vi "Spinner3.vi"(5 "String In":string="sweeping") -> (2 "Spinner Out":string)   [LabVIEW 2019, in "Instrument.Lockin.lvlib" / "Instrument UI.Lockin.lvclass"]
uses:
  Instrument UI.Lockin.lvclass
panel:
  out "s? t:f":i32
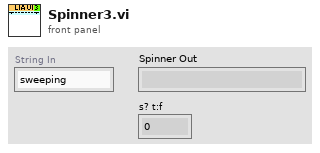
[diagram p1: front panel]
types:
  T1 = enum32{"Bad", "Idle", "Run top level", "Running"}
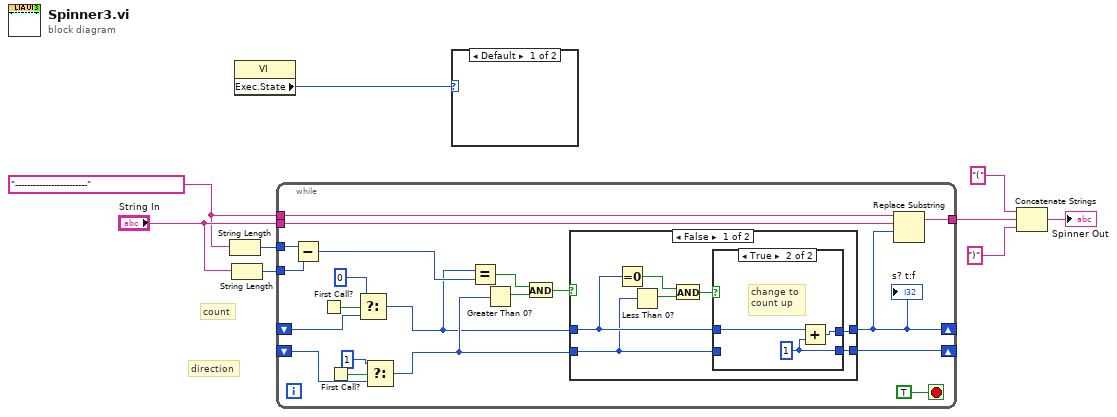
[diagram p0: block diagram]
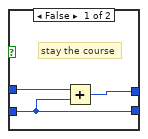
[diagram p2: hidden frame]
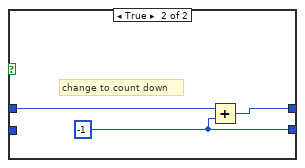
[diagram p3: hidden frame]
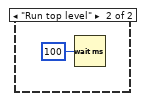
[diagram p4: hidden frame]
diagram:
  w1 = "------------------------"
  # "direction"
  # "count"
  n1 = String Length(string=w1) -> (length=w2:i32)
  n2 = String Length(string="String In") -> (length=w3:i32)
  n3 = property class="VI"() -> ("Exec.State"=w9:T1)  [unwired: 2 in, 2 out]
  n4 = while {
    tunnel: "String In" -> [w28]
    tunnel: w1 -> [w27]
    tunnel: [w26] -> w5
    shift-right: [w10] -> _
    shift-left: _ -> [w13]
    tunnel: w3 -> [w24]
    tunnel: w2 -> [w25]
    shift-right: [w19] -> _
    shift-left: _ -> [w15]
    stop <- TRUE stop-if-true
    n5 = Subtract(x=w25, y=w24) -> (x-y=w23:i32)
    n6 = First Call?() -> (First Call?: T/F=w18:bool)
    n7 = First Call?() -> (First Call?: T/F=w17:bool)
    n8 = Select(t=0 ("y"), s=w18, f=w13) -> (s? t:f=w12:i32)
    n9 = Select(t=1 ("y"), s=w17, f=w15) -> (s? t:f=w14:i32)
    n10 = Equal?(x=w12, y=w23) -> (x = y?=w21:bool)
    n11 = Greater Than 0?(x=w14) -> (x > 0?=w22:bool)
    n12 = And(x=w21, y=w22) -> (x .and. y?=w20:bool)
    n13 = case shown="False" w20 {
      tunnel: w12 -> [w31 w45]
      tunnel: w14 -> [w30 _]
      tunnel: [w32 w43] -> w10
      tunnel: [w33 w44] -> w19
      frame False {
        n14 = Equal To 0?(x=w31) -> (x = 0?=w36:bool)
        n15 = Less Than 0?(x=w30) -> (x < 0?=w35:bool)
        n16 = And(x=w36, y=w35) -> (x .and. y?=w34:bool)
        n17 = case shown="True" w34 {
          tunnel: [w37 w41] -> w33
          tunnel: [w39 w40] -> w32
          tunnel: w31 -> [w38 w42]
          tunnel: w30 -> [w37 _]
          frame False {
            # "stay the course"
            n18 = Add(x=w38, y=w37) -> (x+y=w39:i32)
          }
          frame True {
            w41 = 1 ("y")
            # "change to\ncount up"
            n19 = Add(x=w42, y=w41) -> (x+y=w40:i32)
          }
        }
      }
      frame True {
        w44 = -1 ("y")
        # "change to count down"
        n20 = Add(x=w45, y=w44) -> (x+y=w43:i32)
      }
    }
    "s? t:f" <- w10
    n21 = Replace Substring(3:w10, 4:w28, 5:w27) -> (1:w26:string)  [unwired: 1 in, 1 out]
  }
  n22 = case shown="Default" w9 {
    frame Default {
    }
    frame "Run top level" {
      n23 = Wait (ms)(milliseconds to wait=u32 100) -> ()  [unwired: 1 out]
    }
  }
  n24 = Concatenate Strings("(", w5, ")") -> (→"Spinner Out":string)
